vi "dvp Vi Get Image Data Gray.vi"(0 "handle":u32, 1 "piHeight":i32, 5 "pformat":i32, 7 "pbuffer":u8[](array[numeric])=array[4097 elements], 9 "piWidth":i32, 12 "timeout":u32) -> (3 "piHeight out":i32, 4 "function return":bool, 6 "pformat out":i32, 8 "pbuffer out":u8[](array[numeric]), 10 "piWidth out":i32)   [LabVIEW 2018, in "LabViewDVPCamera.lvlib"]
doc: "LabviewDvp2Api bool dvpViGetImageDataGray(\n dvpHandle handle,\n dvpInt32 *pformat, \n unsigned char pbuffer[],\n dvpInt32 *piWidth,\n dvpInt32 *piHeight, \n dvpUint32 timeout);"
uses:
  LabViewDVPCamera.lvlib
  LabViewDVPCamera/LabViewDVPCamera.dll
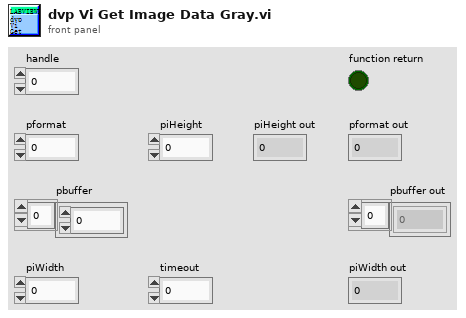
[diagram p1: front panel]
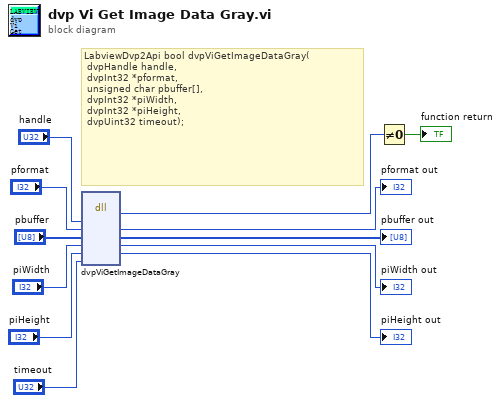
[diagram p0: block diagram]
diagram:
  # "LabviewDvp2Api bool dvpViGetImageDataGray(\n\tdvpHandle handle,\n\tdvpInt32 *pformat, \n\tunsigned char pbuffer[],\n\tdvpInt32 *piWidth,\n\tdvpInt32 *piHeight, \n\tdvpUint32 timeout);"
  n1 = dll-call lib="C:/Program Files (x86)/DVP2 Labview cn 64/Sample/LabViewDVPCamera/LabViewDVPCamera.*" fn="dvpViGetImageDataGray"("handle"="handle", "pformat"="pformat", "pbuffer"="pbuffer", "piWidth"="piWidth", "piHeight"="piHeight", "timeout"="timeout") -> (w11:u8, "pformat"=→"pformat out":i32, "pbuffer"=→"pbuffer out":u8[], "piWidth"=→"piWidth out":i32, "piHeight"=→"piHeight out":i32)  [unwired: 5 in, 2 out]
  n2 = Not Equal To 0?(x=w11) -> (x != 0?=→"function return":bool)
